vi "读取SN码.vi"(8 "error in":errorcluster, 10 "dwLen":u32=16) -> (0 "error out":errorcluster, 1 "return":i32, 2 "SN码":string, 3 "String":string)   [LabVIEW 2016]
panel:
  out "data out":u8[](array[numeric])
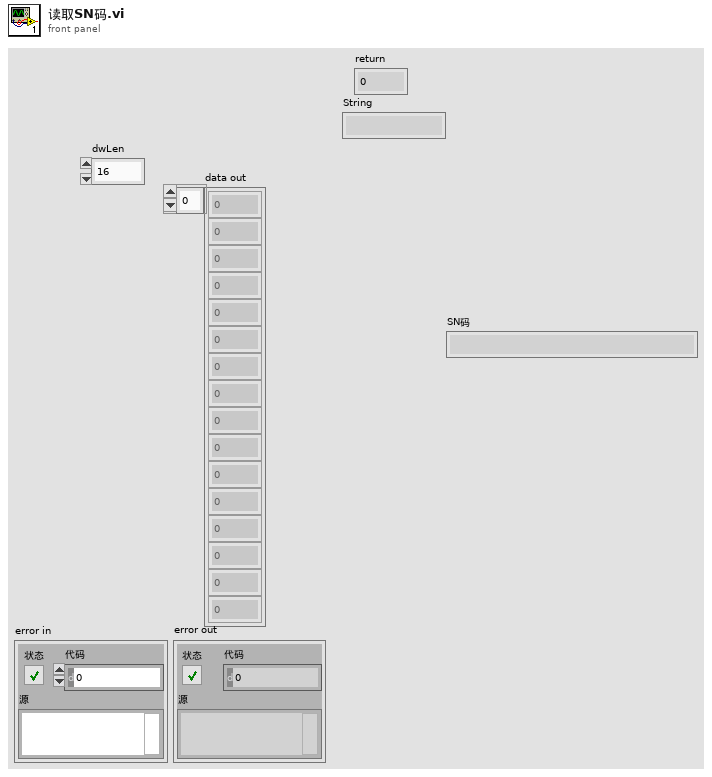
[diagram p1: front panel]
types:
  T1 = cluster{"byCmdType":u8, "bySubCmd":u8, "byPara":u8, "byAddr_h":u8, "byAddr_l":u8, "byAddr_ll":u8, "byLen_h":u8, "byLen_l":u8}
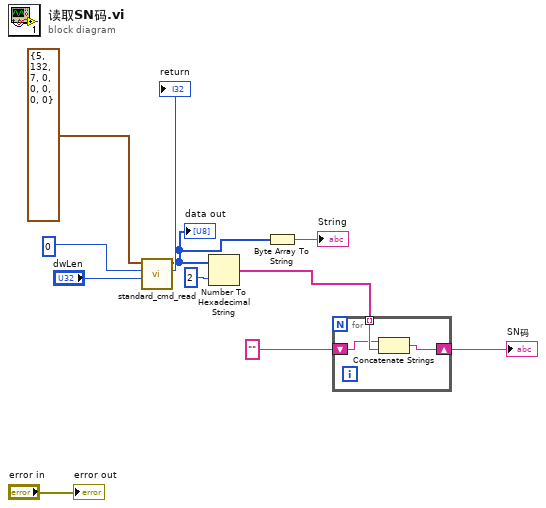
[diagram p0: block diagram]
diagram:
  n1 = call "standard_cmd_read.vi"("dwLen"="dwLen", "dwAddr"=u32 0, "cmd_std_header_t"=T1 {"byCmdType"=5, "bySubCmd"=132, "byPara"=7, "byAddr_h"=0, "byAddr_l"=0, "byAddr_ll"=0, "byLen_h"=0, "byLen_l"=0}) -> ("return"=→"return":i32, "data out"=w2:u8[])  [unwired: 7 in]
  "data out" <- w2
  n2 = Number To Hexadecimal String(1:i16 2 ("width (-)"), 2:w2) -> (0:w3:string[])
  n3 = Byte Array To String(unsigned byte array=w2) -> (string=→"String":string)
  n4 = for {
    shift-right: [w12] -> w5
    shift-left: "" -> [w13]
    tunnel: w3 -> [w14] mode=indexing
    n5 = Concatenate Strings(w13, w14) -> (w12:string)
  }
  "SN码" <- w5
  "error out" <- "error in"
